vi "Do.vi"(8 "error in (no error)":errorcluster, 10 "Actor in":refnum<class "Actor.lvclass">, 11 "Launch Object by Type Msg":refnum<class "Launch Object by Type Msg.lvclass">) -> (0 "error out":errorcluster, 2 "Actor out":refnum<class "Actor.lvclass">)   [LabVIEW 2020, in "Launch Object by Type Msg.lvclass"]
doc: "This VI delivers the message to the actor by calling the appropriate method(s) on the actor."
uses:
  Launch Object by Type Msg.lvclass
  Launch Object by Type Msg.lvclass/Launch Object by Type Msg.ctl
  Application Controller/Application Controller.lvclass
  C:/GitHub/LabActor/Controllers/Process Controller/Process Controller.lvclass
  C:/GitHub/LabActor/Worker/Worker.lvclass
  C:/GitHub/LabActor/Template Module/Template Module.lvclass
  C:/Program Files/National Instruments/LabVIEW 2020/vi.lib/ActorFramework/Actor/Actor.lvclass
  C:/GitHub/LabActor/Controllers/Application Controller/Application Controller.lvclass
  <vilib>/ActorFramework/Actor/Actor.lvclass
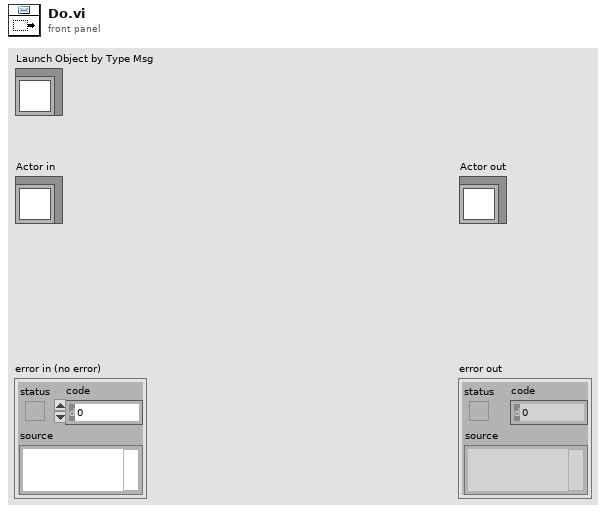
[diagram p1: front panel]
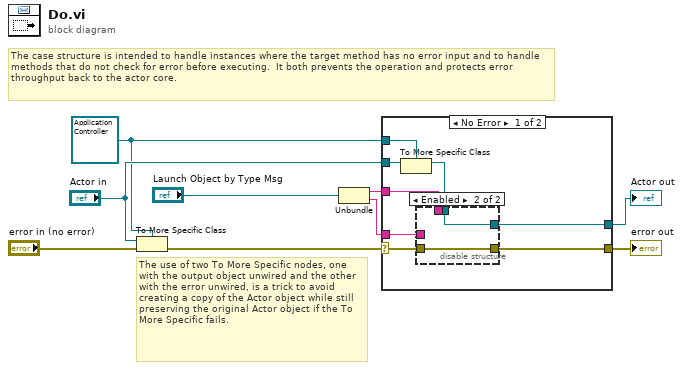
[diagram p0: block diagram]
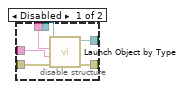
[diagram p2: hidden frame]
diagram:
  w3 = refnum<class "Application Controller.lvclass"> refnum ("Actor in")
  # "The use of two To More Specific nodes, one with the output object unwired and the other with the error unwired, is a trick to avoid creating a copy of the Actor object while still preserving the original Actor object if the To More Specific fails."
  # "The case structure is intended to handle instances where the target method has no error input and to handle methods that do not check for error before executing.  It both prevents the operation and protects error throughput back to the actor core."
  n1 = To More Specific Class(target class=w3, reference="Actor in", error in="error in (no error)") -> (error out=w7:errorcluster)  [unwired: 1 out]
  n2 = Unbundle("Launch Object by Type Msg") -> (w2:string, w1:string)
  n3 = case shown="No Error" w7 {
    selector: w7 -> [w15 w27]
    tunnel: [w17 w27] -> w6
    tunnel: [w16 w26] -> w5
    tunnel: "Actor in" -> [w14 w26]
    tunnel: w3 -> [w13 _]
    tunnel: w2 -> [w11 _]
    tunnel: w1 -> [w10 _]
    frame No Error {
      n4 = To More Specific Class(target class=w13, reference=w14) -> (specific class reference=w12:refnum<class "Application Controller.lvclass">)  [unwired: 1 in, 1 out]
      n5 = disable-structure shown="Enabled" {
        disable-tunnel: [w23 w24] -> w17
        disable-tunnel: [w22 w25] -> w16
        disable-tunnel: w15 -> [w21 w24]
        disable-tunnel: w12 -> [w20 w25]
        disable-tunnel: w11 -> [w19 _]
        disable-tunnel: w10 -> [w18 _]
        frame Disabled {
          n6 = call-dynamic "Launch Object by Type.vi"("error in (no error)"=w21, "Requestor"=w18, "Type"=w19, "Application Controller in"=w20) -> ("error out"=w23:errorcluster, "Application Controller out"=w22:refnum<class "Application Controller.lvclass">)  [unwired: 6 in]
        }
        frame Enabled {
        }
      }
    }
    frame Error {
      # "If type check fails, pass the original object out again."
    }
  }
  "error out" <- w6
  "Actor out" <- w5
